vi "GetVersionSerializableData.vi"(10 "Version":u16, 11 "Golf Club":refnum<class "Golf Club.lvclass">) -> (0 "error out":errorcluster, 1 "Found?":bool, 2 "SerializableData":variant, 3 "Golf Club":refnum<class "Golf Club.lvclass">)   [LabVIEW 2019, in "Golf Club.lvclass"]
uses:
  Golf Club.lvclass
  SerializableData_v1.ctl
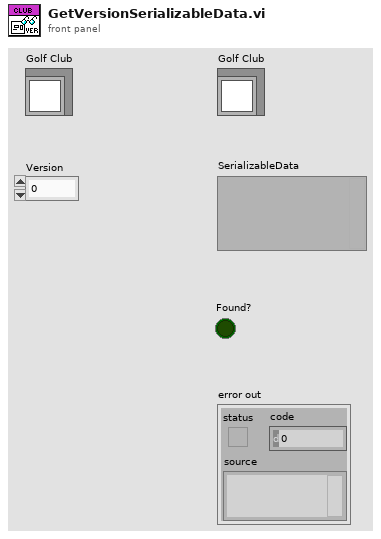
[diagram p1: front panel]
types:
  T1 = typedef "Golf Club.lvclass/SerializableData_v1.ctl" = cluster{"Club Number":i32}
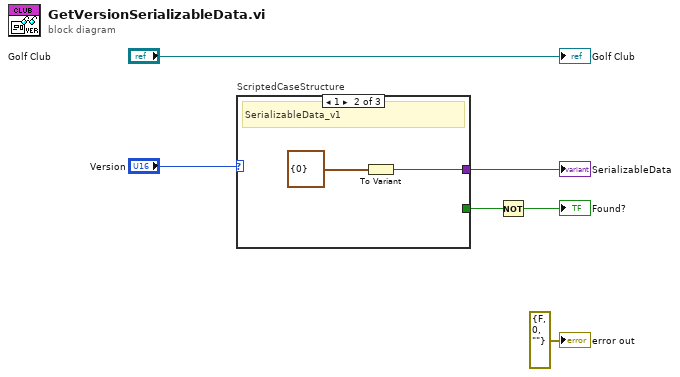
[diagram p0: block diagram]
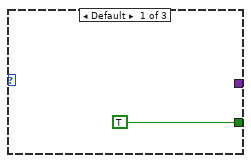
[diagram p2: hidden frame]
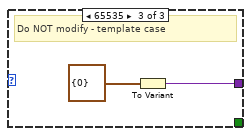
[diagram p3: hidden frame]
diagram:
  n1 = case "ScriptedCaseStructure" shown="1" "Version" {
    tunnel: [_ w9 w11] -> w5
    tunnel: [TRUE _ _] -> w4
    frame Default {
    }
    frame 1 {
      # "SerializableData_v1"
      n2 = To Variant(anything=T1 {"Club Number"=0} ("SerializableData")) -> (Variant=w9:variant)
    }
    frame 65535 {
      # "Do NOT modify - template case"
      n3 = To Variant(anything=T1 {"Club Number"=0} ("SerializableData")) -> (Variant=w11:variant)
    }
  }
  "SerializableData" <- w5
  n4 = Not(x=w4) -> (.not. x?=→"Found?":bool)
  "error out" <- errorcluster {"status"=FALSE, "code"=0, "source"=""} ("error out")
  "Golf Club" <- "Golf Club"
